vi "Bool Collor control.vi"(4 "NG":u32(colorbox)=16711680, 5 "OK":u32(colorbox)=4390811, 6 "Color":cluster{"Initialize":u32, "Testing":u32}={"Initialize"=0, "Testing"=16383786}, 7 "Result":T1(ring), 8 "error in (no error)":errorcluster, 9 "BoolText":string, 10 "Value":bool, 11 "Bool Refnum":refnum<vi>) -> (0 "error out":errorcluster, 3 "reference out":refnum<vi>)   [LabVIEW 2021]
panel:
  in  "Colors [4]":cluster{"Color Box":u32, "Color Box 2":u32}[](array[cluster])=[{"Color Box"=4671303, "Color Box 2"=4671303}, {"Color Box"=16734592, "Color Box 2"=4390811}, {"Color Box"=2302755, "Color Box 2"=2302755}, {"Color Box"=2195277, "Color Box 2"=2195277}]
  in  "s":bool
  out "Boolean":bool
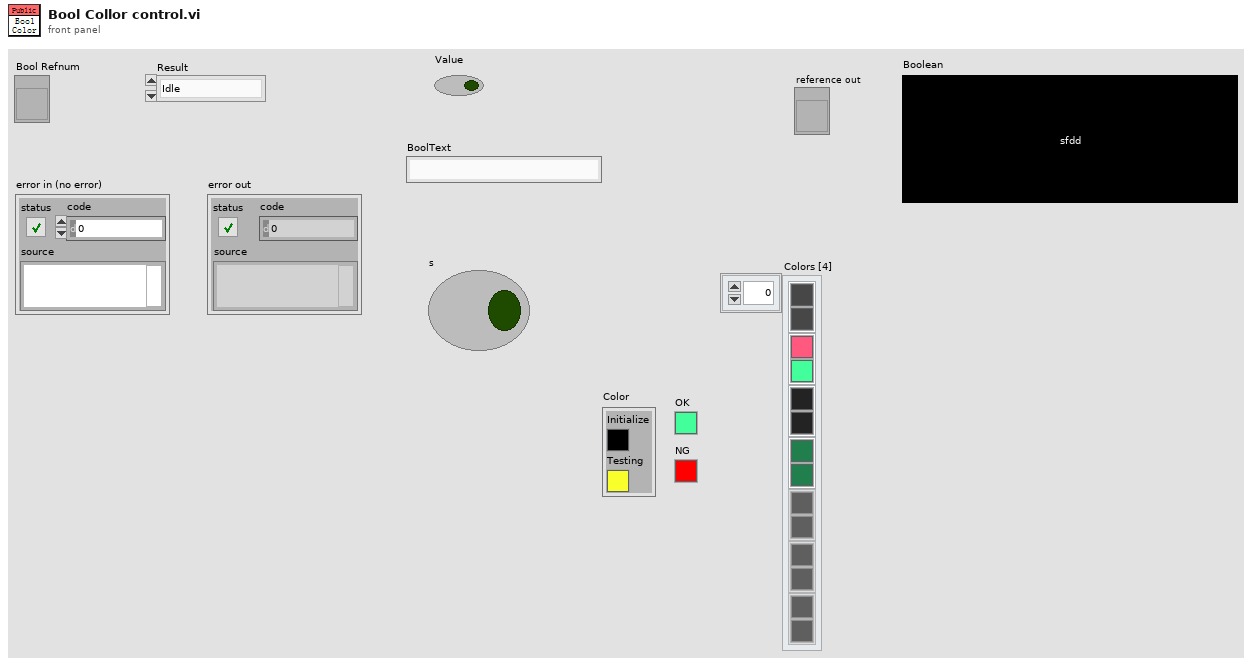
[diagram p1: front panel]
types:
  T1 = enum16{"Idle", "Initialzie", "Testing", "OK", "NG"}
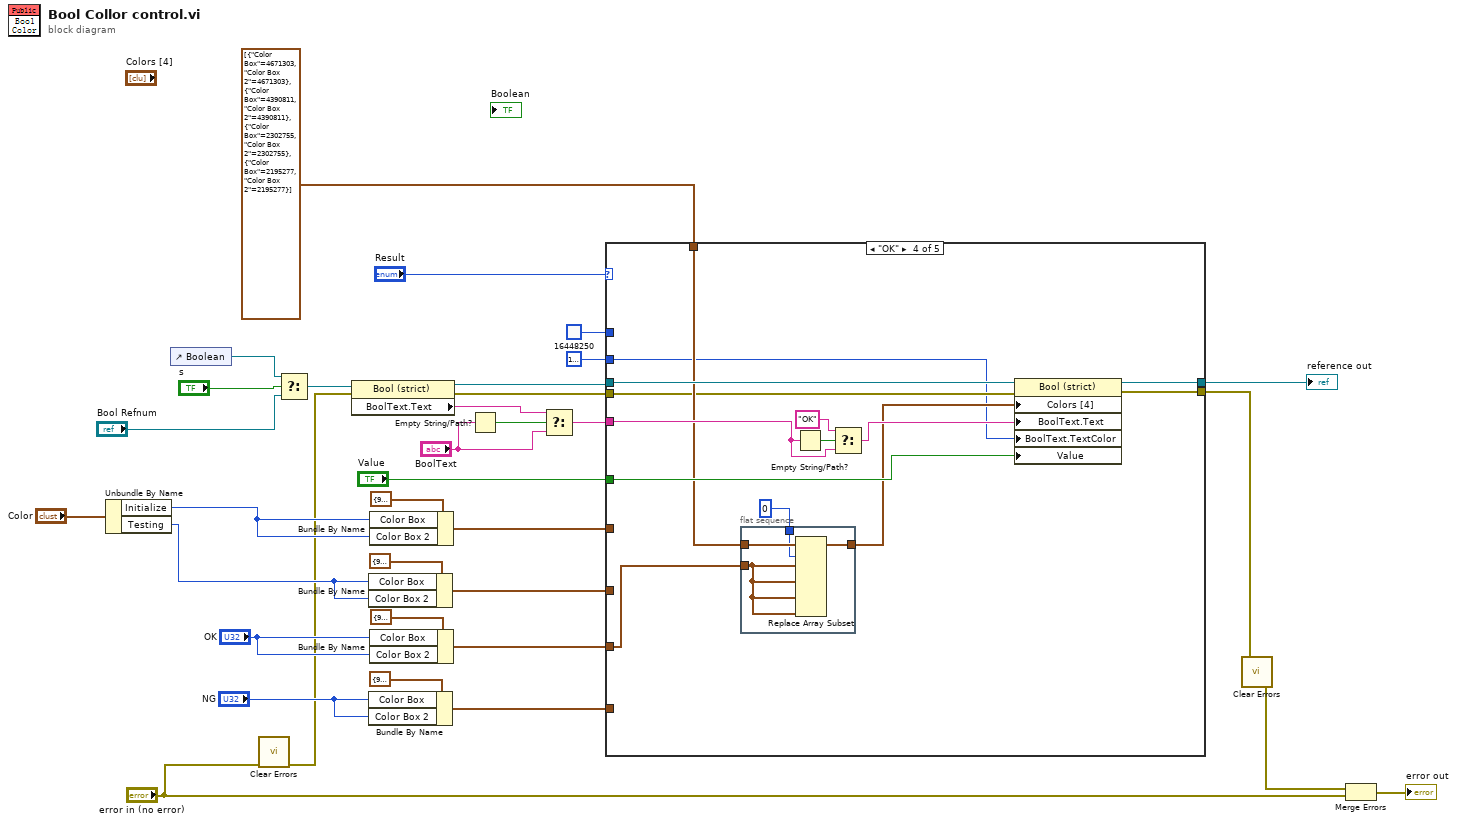
[diagram p0: block diagram]
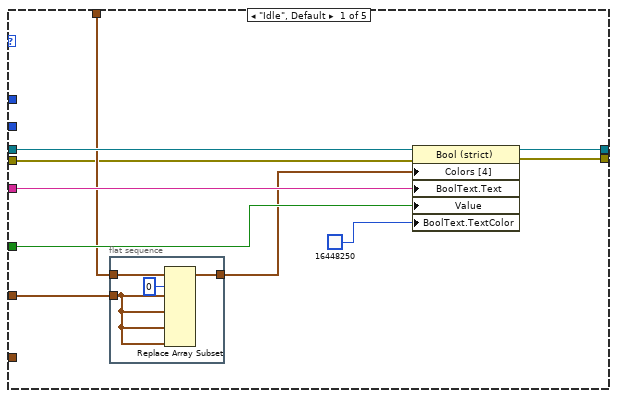
[diagram p2: hidden frame]
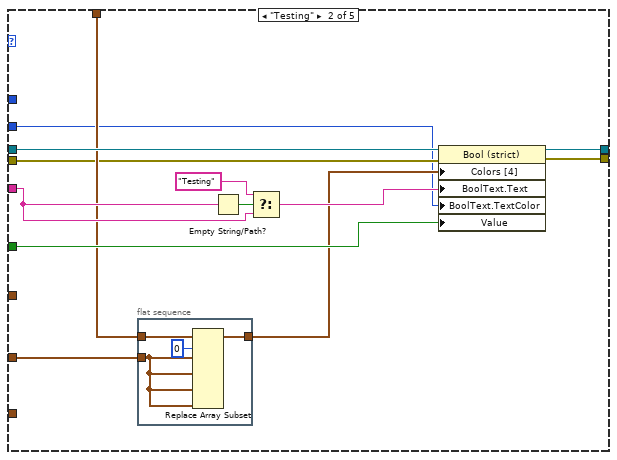
[diagram p3: hidden frame]
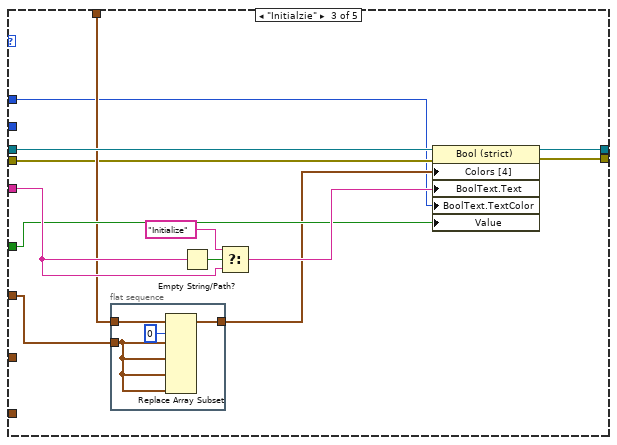
[diagram p4: hidden frame]
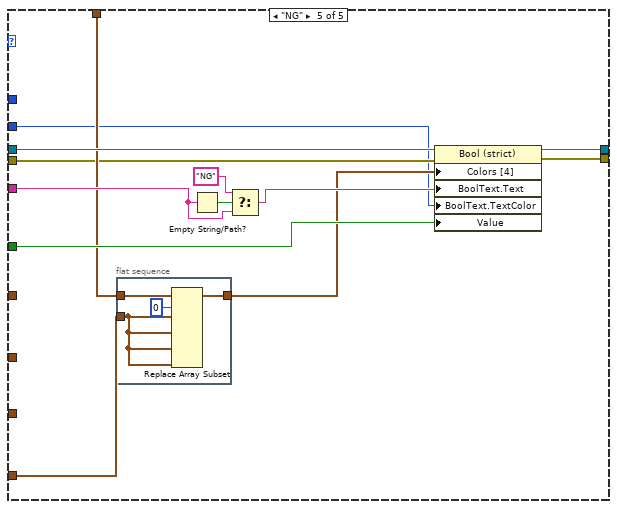
[diagram p5: hidden frame]
diagram:
  n1 = Unbundle By Name("Color") -> ("Initialize"=w11:u32, "Testing"=w10:u32)
  n2 = control-ref of="Boolean"() -> (w31:refnum<vi>)
  n3 = call <vilib>:"Clear Errors.vi"("error in (no error)"="error in (no error)") -> ("error out"=w4:errorcluster)  [unwired: 5 in, 1 out]
  n4 = Select(t=w31, s="s", f="Bool Refnum") -> (s? t:f=w28:refnum<vi>)
  n5 = property class="Bool (strict)"(reference=w28, error in=w4) -> (reference out=w25:refnum<vi>, error out=w7:errorcluster, "BoolText.Text"=w33:string)
  n6 = Bundle By Name(cluster=cluster{"Color Box":u32, "Color Box 2":u32} {"Color Box"=9868950, "Color Box 2"=9868950} ("Cluster"), "Color Box"=w10, "Color Box 2"=w10) -> (w16:cluster{"Color Box":u32, "Color Box 2":u32})
  n7 = Bundle By Name(cluster=cluster{"Color Box":u32, "Color Box 2":u32} {"Color Box"=9868950, "Color Box 2"=9868950} ("Cluster"), "Color Box"="NG", "Color Box 2"="NG") -> (w18:cluster{"Color Box":u32, "Color Box 2":u32})
  n8 = Bundle By Name(cluster=cluster{"Color Box":u32, "Color Box 2":u32} {"Color Box"=9868950, "Color Box 2"=9868950} ("Cluster"), "Color Box"=w11, "Color Box 2"=w11) -> (w14:cluster{"Color Box":u32, "Color Box 2":u32})
  n9 = Bundle By Name(cluster=cluster{"Color Box":u32, "Color Box 2":u32} {"Color Box"=9868950, "Color Box 2"=9868950} ("Cluster"), "Color Box"="OK", "Color Box 2"="OK") -> (w21:cluster{"Color Box":u32, "Color Box 2":u32})
  n10 = Empty String/Path?(string/path="BoolText") -> (empty?=w34:bool)
  n11 = Select(t=w33, s=w34, f="BoolText") -> (s? t:f=w26:string)
  n12 = case shown="\"OK\"" "Result" {
    tunnel: w25 -> [w43 w60 w77 w95 w112]
    tunnel: w26 -> [w44 w59 w76 w94 w111]
    tunnel: "Value" -> [w42 w56 w73 w91 w108]
    tunnel: w21 -> [_ _ _ w90 _]
    tunnel: w18 -> [_ _ _ _ w107]
    tunnel: cluster{"Color Box":u32, "Color Box 2":u32}[] [{"Color Box"=4671303, "Color Box 2"=4671303}, {"Color Box"=4390811, "Color Box 2"=4390811}, {"Color Box"=2302755, "Color Box 2"=2302755}, {"Color Box"=2195277, "Color Box 2"=2195277}] ("Colors [4]") -> [w41 w54 w71 w89 w106]
    tunnel: w14 -> [w39 _ w72 _ _]
    tunnel: w16 -> [_ w55 _ _ _]
    tunnel: w7 -> [w38 w52 w69 w87 w104]
    tunnel: [w37 w51 w68 w86 w103] -> w6
    tunnel: u32 16777222 ("Color Box") -> [_ w50 _ w85 w102]
    tunnel: u32 16448250 ("Color Box") -> [_ _ w67 _ _]
    tunnel: [w35 w49 w66 w84 w101] -> w1
    frame "Idle", Default {
      n13 = flat-sequence {
        tunnel: w41 -> [w48]
        tunnel: [w46] -> w40
        tunnel: w39 -> [w45]
        frame #0 {
          n14 = Replace Array Subset(array=w48, new element #1=w45, index #1=0 ("index"), new element #2=w45, new element #3=w45, new element #4=w45) -> (w46:cluster{"Color Box":u32, "Color Box 2":u32}[])  [unwired: 3 in]
        }
      }
      n15 = property class="Bool (strict)"(reference=w43, error in=w38, "Colors [4]"=w40, "BoolText.Text"=w44, "Value"=w42, "BoolText.TextColor"=u32 16448250 ("Color Box")) -> (reference out=w35:refnum<vi>, error out=w37:errorcluster)
    }
    frame "Testing" {
      n16 = flat-sequence {
        tunnel: w54 -> [w65]
        tunnel: [w63] -> w53
        tunnel: w55 -> [w62]
        frame #0 {
          n17 = Replace Array Subset(array=w65, new element #1=w62, index #1=0 ("index"), new element #2=w62, new element #3=w62, new element #4=w62) -> (w63:cluster{"Color Box":u32, "Color Box 2":u32}[])  [unwired: 3 in]
        }
      }
      n18 = Empty String/Path?(string/path=w59) -> (empty?=w58:bool)
      n19 = Select(t="Testing", s=w58, f=w59) -> (s? t:f=w61:string)
      n20 = property class="Bool (strict)"(reference=w60, error in=w52, "Colors [4]"=w53, "BoolText.Text"=w61, "BoolText.TextColor"=w50, "Value"=w56) -> (reference out=w49:refnum<vi>, error out=w51:errorcluster)
    }
    frame "Initialzie" {
      n21 = flat-sequence {
        tunnel: w71 -> [w82]
        tunnel: [w80] -> w70
        tunnel: w72 -> [w79]
        frame #0 {
          n22 = Replace Array Subset(array=w82, new element #1=w79, index #1=0 ("index"), new element #2=w79, new element #3=w79, new element #4=w79) -> (w80:cluster{"Color Box":u32, "Color Box 2":u32}[])  [unwired: 3 in]
        }
      }
      n23 = Empty String/Path?(string/path=w76) -> (empty?=w75:bool)
      n24 = Select(t="Initialize" ("BoolText 2"), s=w75, f=w76) -> (s? t:f=w78:string)
      n25 = property class="Bool (strict)"(reference=w77, error in=w69, "Colors [4]"=w70, "BoolText.Text"=w78, "BoolText.TextColor"=w67, "Value"=w73) -> (reference out=w66:refnum<vi>, error out=w68:errorcluster)
    }
    frame "OK" {
      n26 = flat-sequence {
        tunnel: w89 -> [w100]
        tunnel: [w99] -> w88
        tunnel: w90 -> [w98]
        tunnel: 0 ("index") -> [w97]
        frame #0 {
          n27 = Replace Array Subset(array=w100, new element #1=w98, index #1=w97, new element #2=w98, new element #3=w98, new element #4=w98) -> (w99:cluster{"Color Box":u32, "Color Box 2":u32}[])  [unwired: 3 in]
        }
      }
      n28 = Empty String/Path?(string/path=w94) -> (empty?=w93:bool)
      n29 = Select(t="OK", s=w93, f=w94) -> (s? t:f=w96:string)
      n30 = property class="Bool (strict)"(reference=w95, error in=w87, "Colors [4]"=w88, "BoolText.Text"=w96, "BoolText.TextColor"=w85, "Value"=w91) -> (reference out=w84:refnum<vi>, error out=w86:errorcluster)
    }
    frame "NG" {
      n31 = flat-sequence {
        tunnel: w106 -> [w117]
        tunnel: [w115] -> w105
        tunnel: w107 -> [w114]
        frame #0 {
          n32 = Replace Array Subset(array=w117, new element #1=w114, index #1=0 ("index"), new element #2=w114, new element #3=w114, new element #4=w114) -> (w115:cluster{"Color Box":u32, "Color Box 2":u32}[])  [unwired: 3 in]
        }
      }
      n33 = Empty String/Path?(string/path=w111) -> (empty?=w110:bool)
      n34 = Select(t="NG", s=w110, f=w111) -> (s? t:f=w113:string)
      n35 = property class="Bool (strict)"(reference=w112, error in=w104, "Colors [4]"=w105, "BoolText.Text"=w113, "BoolText.TextColor"=w102, "Value"=w108) -> (reference out=w101:refnum<vi>, error out=w103:errorcluster)
    }
  }
  "reference out" <- w1
  n36 = call <vilib>:"Clear Errors.vi"("error in (no error)"=w6) -> ("error out"=w5:errorcluster)  [unwired: 5 in, 1 out]
  n37 = Merge Errors(w5, "error in (no error)") -> (→"error out":errorcluster)
